vi "PXI-Get Terminal Configuration.vi"(7 "term config in":i32(ring)=-1 items=["Default"=-1, "RSE"=10083, "NRSE"=10078, "Differential"=10106, "Pseudodifferential"=12529], 11 "error in (no error)":errorcluster, 13 "channel":string) -> (8 "term config out":i32(ring)=-1 items=["Default"=-1, "RSE"=10083, "NRSE"=10078, "Differential"=10106, "Pseudodifferential"=12529], 15 "error out":errorcluster)   [LabVIEW 2020]
uses:
  <vilib>/Utility/config.llb/Read Key (String).vi
  <vilib>/Utility/config.llb/NI_LVConfig.lvlib
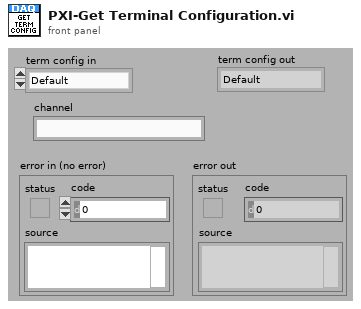
[diagram p1: front panel]
types:
  T1 = typedef "LVStringsAndValuesArrayTypeDef_I32.ctl" = cluster{"String":string, "Value":i32}[]
  T2 = typedef "NI_LVConfig.lvlib/Config Data RefNum.ctl" = refnum<k1>
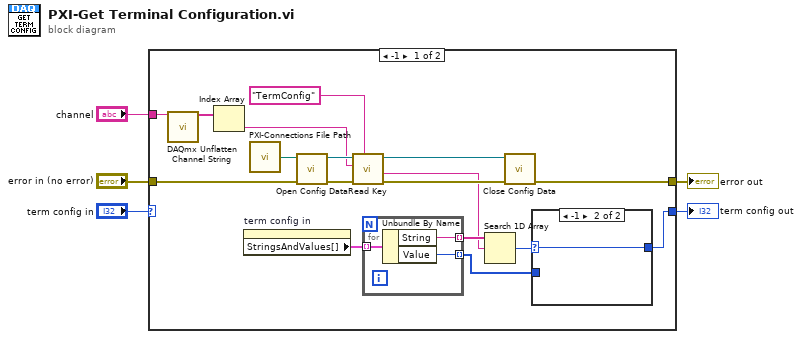
[diagram p0: block diagram]
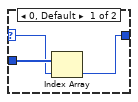
[diagram p2: hidden frame]
diagram:
  n1 = case shown="-1" "term config in" {
    selector: "term config in" -> [_ w31]
    tunnel: "error in (no error)" -> [w22 w30]
    tunnel: [w16 w30] -> w4
    tunnel: [w10 w31] -> w2
    tunnel: "channel" -> [w8 _]
    frame -1 {
      n2 = call <vilib>:"DAQmx Unflatten Channel String.vi"("names in"=w8) -> ("names out"=w7:string[])  [unwired: 13 in, 1 out]
      n3 = Index Array(array=w7) -> (element=w6:string)  [unwired: 1 in]
      n4 = property on="term config in" class="Ring (strict)"() -> ("StringsAndValues[]"=w14:T1)  [unwired: 2 in, 2 out]
      n5 = call "PXI-Connections File Path.vi"() -> ("Path"=w15:path)  [unwired: 1 in]
      n6 = call <vilib>:"Open Config Data.vi"("error in (no error)"=w22, "configuration file path"=w15) -> ("error out"=w21:errorcluster, "refnum"=w20:T2)  [unwired: 7 in, 1 out]
      n7 = call-poly <vilib>:"Read Key.vi"("section"="TermConfig", "error in (no error)"=w21, "key"=w6, "refnum"=w20) -> ("error out"=w18:errorcluster, "value"=w12:string, "refnum out"=w17:T2)  [unwired: 4 in, 1 out]
      n8 = for {
        tunnel: w14 -> [w29] mode=indexing
        tunnel: [w28] -> w13 mode=indexing
        tunnel: [w27] -> w9 mode=indexing
        n9 = Unbundle By Name(w29) -> ("String"=w28:string, "Value"=w27:i32)
      }
      n10 = Search 1D Array(1D array=w13, element=w12) -> (index of element=w11:i32)  [unwired: 1 in]
      n11 = call <vilib>:"Close Config Data.vi"("error in (no error)"=w18, "refnum"=w17) -> ("error out"=w16:errorcluster)  [unwired: 8 in, 1 out]
      n12 = case shown="-1" w11 {
        selector: w11 -> [w24 w26]
        tunnel: [w23 w26] -> w10
        tunnel: w9 -> [w25 _]
        frame 0, Default {
          n13 = Index Array(array=w25, index=w24) -> (element=w23:i32)
        }
        frame -1 {
        }
      }
    }
    frame 1, Default {
    }
  }
  "error out" <- w4
  "term config out" <- w2
